vi "Wolna_rozdziel_buf.vi"(8 "error in (no error)":errorcluster, 9 "Data in":T1, 10 "bufor OK in":bool, 11 "Okres in":dbl) -> (0 "error out":errorcluster, 1 "Data out":T1, 2 "bufor OK out":bool, 3 "Wydzielone out":T1)   [LabVIEW 2013]
doc: "Jeżeli bufor jest OK\nto rozdziela na dane do obliczenia i resztę buforu"
uses:
  Kontrolki/Przetwarzanie/Kanaly.ctl
panel:
  in  "#cores (1)":i32=1
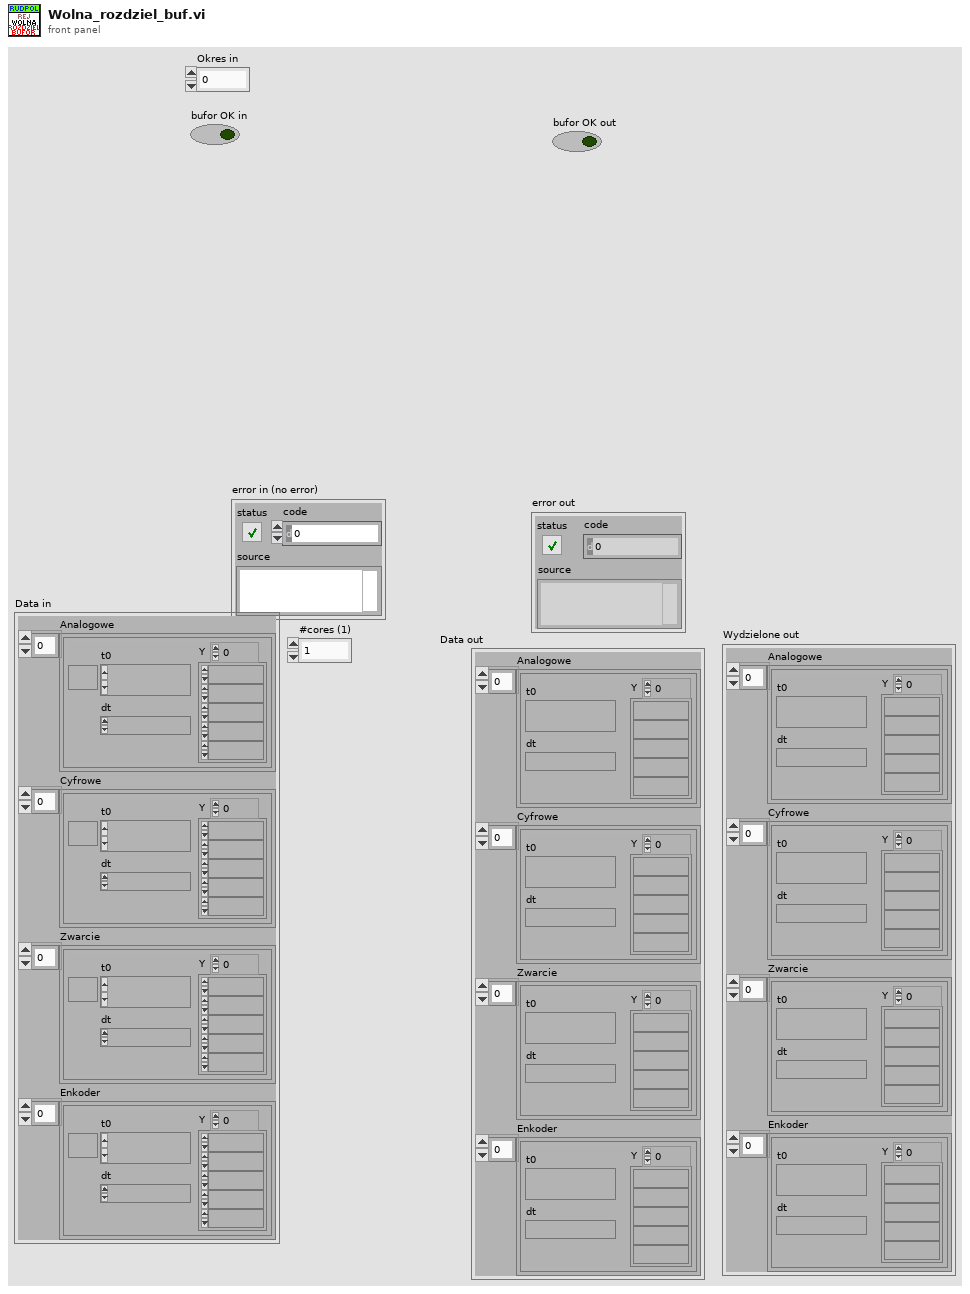
[diagram p1: front panel]
types:
  T1 = typedef "Kanaly.ctl" = cluster{"Analogowe":waveform(dbl)[], "Cyfrowe":waveform(dbl)[], "Zwarcie":waveform(dbl)[], "Enkoder":waveform(dbl)[]}
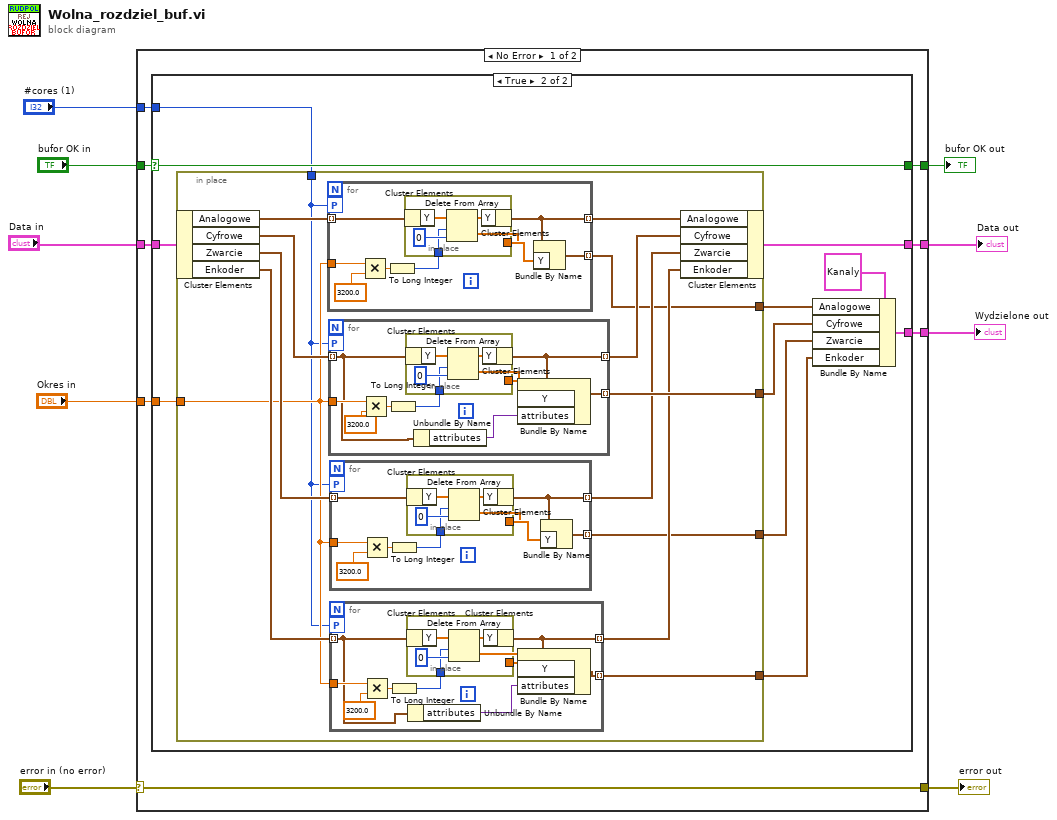
[diagram p0: block diagram]
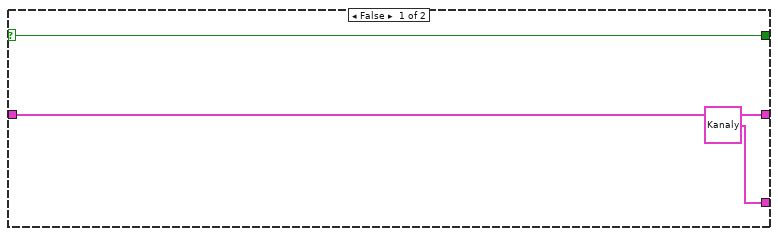
[diagram p2: hidden frame]
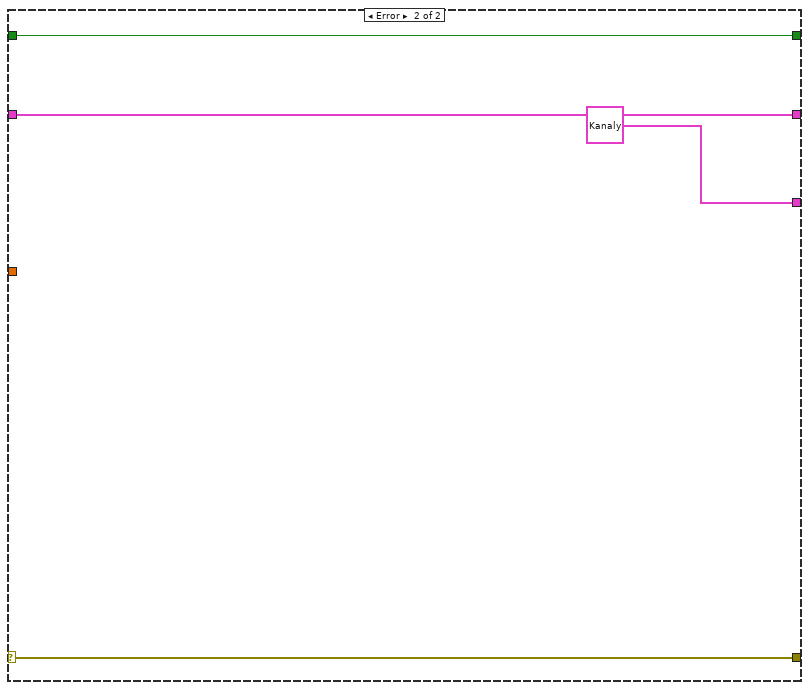
[diagram p3: hidden frame]
diagram:
  n1 = case shown="No Error" "error in (no error)" {
    selector: "error in (no error)" -> [w11 w102]
    tunnel: "Okres in" -> [w17 _]
    tunnel: "Data in" -> [w16 w101]
    tunnel: "bufor OK in" -> [w15 w103]
    tunnel: [w14 w101] -> w3
    tunnel: [w13 T1 data[32432B] ("Data in 2")] -> w2
    tunnel: [w12 w103] -> w7
    tunnel: [w11 w102] -> w5
    tunnel: "#cores (1)" -> [w10 _]
    frame No Error {
      n2 = case shown="True" w15 {
        selector: w15 -> [w20 w31]
        tunnel: w16 -> [w19 w26]
        tunnel: [w19 w29] -> w14
        tunnel: [w20 w31] -> w12
        tunnel: w17 -> [_ w30]
        tunnel: [T1 data[32432B] ("Data in 2") w27] -> w13
        tunnel: w10 -> [_ w21]
        frame False {
        }
        frame True {
          n3 = in-place {
            in-place-border: w30 -> [w38]
            in-place-border: [w43] -> w25
            in-place-border: [w35] -> w24
            in-place-border: [w34] -> w23
            in-place-border: [w33] -> w22
            in-place-border: w21 -> [w32]
            n4 = in-place-cluster #1(w26) -> ("Analogowe"=w45:waveform(dbl)[], "Cyfrowe"=w42:waveform(dbl)[], "Zwarcie"=w40:waveform(dbl)[], "Enkoder"=w39:waveform(dbl)[])
            n5 = for {
              tunnel: w38 -> [w92]
              tunnel: [w88] -> w44 mode=indexing
              tunnel: [w91] -> w35 mode=indexing
              tunnel: w45 -> [w87] mode=indexing
              workers-P: w32 -> [_]
              n6 = Multiply(x=w92, y=3200.0) -> (x*y=w94:dbl)
              n7 = To Long Integer(number=w94) -> (32bit integer=w90:i32)
              n8 = in-place {
                in-place-border: w90 -> [w96]
                in-place-border: [w95] -> w89
                n9 = in-place-cluster #2(w87) -> ("Y"=w99:dbl[])
                n10 = Delete From Array(array=w99, length=w96, index=0) -> (deleted portion=w95:dbl[], array with subset deleted=w98:dbl[])
                n11 = in-place-cluster #2("Y"=w98) -> (w88:waveform(dbl))
              }
              n12 = Bundle By Name(cluster=w88, "Y"=w89) -> (w91:waveform(dbl))
            }
            n13 = for {
              tunnel: [w76] -> w41 mode=indexing
              tunnel: [w79] -> w43 mode=indexing
              tunnel: w42 -> [w73] mode=indexing
              tunnel: w38 -> [w75]
              workers-P: w32 -> [_]
              n14 = Multiply(x=w75, y=3200.0) -> (x*y=w81:dbl)
              n15 = To Long Integer(number=w81) -> (32bit integer=w78:i32)
              n16 = in-place {
                in-place-border: w78 -> [w83]
                in-place-border: [w82] -> w77
                n17 = in-place-cluster #3(w73) -> ("Y"=w86:dbl[])
                n18 = Delete From Array(array=w86, length=w83, index=0) -> (deleted portion=w82:dbl[], array with subset deleted=w85:dbl[])
                n19 = in-place-cluster #3("Y"=w85) -> (w76:waveform(dbl))
              }
              n20 = Unbundle By Name(w73) -> ("attributes"=w74:variant)
              n21 = Bundle By Name(cluster=w76, "Y"=w77, "attributes"=w74) -> (w79:waveform(dbl))
            }
            n22 = for {
              tunnel: [w62] -> w37 mode=indexing
              tunnel: [w65] -> w34 mode=indexing
              tunnel: w40 -> [w61] mode=indexing
              tunnel: w38 -> [w60]
              workers-P: w32 -> [_]
              n23 = Multiply(x=w60, y=3200.0) -> (x*y=w67:dbl)
              n24 = To Long Integer(number=w67) -> (32bit integer=w64:i32)
              n25 = in-place {
                in-place-border: w64 -> [w69]
                in-place-border: [w68] -> w63
                n26 = in-place-cluster #4(w61) -> ("Y"=w72:dbl[])
                n27 = Delete From Array(array=w72, length=w69, index=0) -> (deleted portion=w68:dbl[], array with subset deleted=w71:dbl[])
                n28 = in-place-cluster #4("Y"=w71) -> (w62:waveform(dbl))
              }
              n29 = Bundle By Name(cluster=w62, "Y"=w63) -> (w65:waveform(dbl))
            }
            n30 = for {
              tunnel: [w49] -> w36 mode=indexing
              tunnel: [w52] -> w33 mode=indexing
              tunnel: w39 -> [w46] mode=indexing
              tunnel: w38 -> [w48]
              workers-P: w32 -> [_]
              n31 = Multiply(x=w48, y=3200.0) -> (x*y=w54:dbl)
              n32 = To Long Integer(number=w54) -> (32bit integer=w51:i32)
              n33 = in-place {
                in-place-border: w51 -> [w56]
                in-place-border: [w55] -> w50
                n34 = in-place-cluster #5(w46) -> ("Y"=w59:dbl[])
                n35 = Delete From Array(array=w59, length=w56, index=0) -> (deleted portion=w55:dbl[], array with subset deleted=w58:dbl[])
                n36 = in-place-cluster #5("Y"=w58) -> (w49:waveform(dbl))
              }
              n37 = Unbundle By Name(w46) -> ("attributes"=w47:variant)
              n38 = Bundle By Name(cluster=w49, "Y"=w50, "attributes"=w47) -> (w52:waveform(dbl))
            }
            n39 = in-place-cluster #1("Analogowe"=w44, "Cyfrowe"=w41, "Zwarcie"=w37, "Enkoder"=w36) -> (w29:T1)
          }
          n40 = Bundle By Name(cluster=T1 data[32432B] ("Data in 2"), "Analogowe"=w24, "Cyfrowe"=w25, "Zwarcie"=w23, "Enkoder"=w22) -> (w27:T1)
        }
      }
    }
    frame Error {
    }
  }
  "bufor OK out" <- w7
  "error out" <- w5
  "Data out" <- w3
  "Wydzielone out" <- w2
